vi "3.1.vi"(0 "x":dbl) -> (1 "z":dbl, 2 "y":dbl)   [LabVIEW 2017]
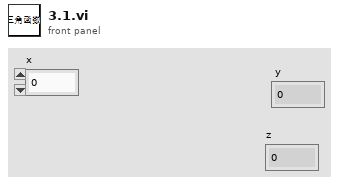
[diagram p1: front panel]
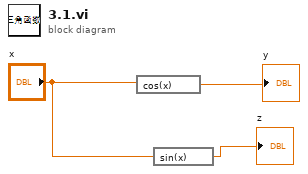
[diagram p0: block diagram]
diagram:
  n1 = expression code="cos(x)"("x") -> (→"y":dbl)
  n2 = expression code="sin(x)"("x") -> (→"z":dbl)
